vi "CRYConstant Arithmetic Operation.vi"(4 "Constant":dbl, 6 "B data for units":T1={"Name"="", "Curve"=[], "X data"=1, "Y data"=1, "Z data"=1, "X axis"=0, "Y axis"=1, "Z axis"=1, "X unit"="Hz", "Y unit"="", "Z unit"="deg.", "X dB ref"=1.0, "Y dB ref"=1.0, "Z dB ref"=1.0, "single val"=FALSE, "protected"=FALSE, "display X"=TRUE, "display Y"=TRUE, "display Z"=TRUE, "Test Info"="", "Step No."=0, "Plot Settings"={"Color"=0, "Interpolation"=0, "Point Style"=0, "Line Style"=0, "Point Color"=0, "Line Width"=0, "Bar Plot Style"=0, "Fill To"=0}, "AutoProtect"=FALSE} {"Z data" items=["dB", "Lin"]; "X data" items=["dB", "Lin"]; "Y data" items=["dB", "Lin"]; "Z dB ref" format="%.1f"; "Z axis" items=["Log", "Lin"]; "X dB ref" format="%.1f"; "X axis" items=["Log", "Lin"]; "Y axis" items=["Log", "Lin"]; "Y dB ref" format="%.1f"; "Curve"."z" format="%.2f"; "Curve"."y" format="%.2f"; "Curve"."x" format="%.2f"}, 7 "A data for units":T1={"Name"="", "Curve"=[], "X data"=1, "Y data"=1, "Z data"=1, "X axis"=0, "Y axis"=1, "Z axis"=1, "X unit"="Hz", "Y unit"="", "Z unit"="deg.", "X dB ref"=1.0, "Y dB ref"=1.0, "Z dB ref"=1.0, "single val"=FALSE, "protected"=FALSE, "display X"=TRUE, "display Y"=TRUE, "display Z"=TRUE, "Test Info"="", "Step No."=0, "Plot Settings"={"Color"=0, "Interpolation"=0, "Point Style"=0, "Line Style"=0, "Point Color"=0, "Line Width"=0, "Bar Plot Style"=0, "Fill To"=0}, "AutoProtect"=FALSE} {"Z data" items=["dB", "Lin"]; "X data" items=["dB", "Lin"]; "Y data" items=["dB", "Lin"]; "Z dB ref" format="%.1f"; "Z axis" items=["Log", "Lin"]; "X dB ref" format="%.1f"; "X axis" items=["Log", "Lin"]; "Y axis" items=["Log", "Lin"]; "Y dB ref" format="%.1f"; "Curve"."z" format="%.2f"; "Curve"."y" format="%.2f"; "Curve"."x" format="%.2f"}, 8 "B_axis mode":u16(slide) scale=0.0..2.0, 9 "A_axis mode":u16(slide) scale=0.0..2.0, 10 "Work in":u16(slide), 11 "Operator":u16(ring) items=["+", "--", "x", "/"]) -> (3 "Result out":T1={"Name"="", "Curve"=[], "X data"=1, "Y data"=1, "Z data"=1, "X axis"=0, "Y axis"=1, "Z axis"=1, "X unit"="Hz", "Y unit"="", "Z unit"="deg.", "X dB ref"=1.0, "Y dB ref"=1.0, "Z dB ref"=1.0, "single val"=FALSE, "protected"=FALSE, "display X"=TRUE, "display Y"=TRUE, "display Z"=TRUE, "Test Info"="", "Step No."=0, "Plot Settings"={"Color"=0, "Interpolation"=0, "Point Style"=0, "Line Style"=0, "Point Color"=0, "Line Width"=0, "Bar Plot Style"=0, "Fill To"=0}, "AutoProtect"=FALSE} {"Z data" items=["dB", "Lin"]; "X data" items=["dB", "Lin"]; "Y data" items=["dB", "Lin"]; "Z dB ref" format="%.1f"; "Z axis" items=["Log", "Lin"]; "X dB ref" format="%.1f"; "X axis" items=["Log", "Lin"]; "Y axis" items=["Log", "Lin"]; "Y dB ref" format="%.1f"; "Curve"."z" format="%.2f"; "Curve"."y" format="%.2f"; "Curve"."x" format="%.2f"})   [LabVIEW 2013]
uses:
  Typedef Control/CRYData Cluster.ctl
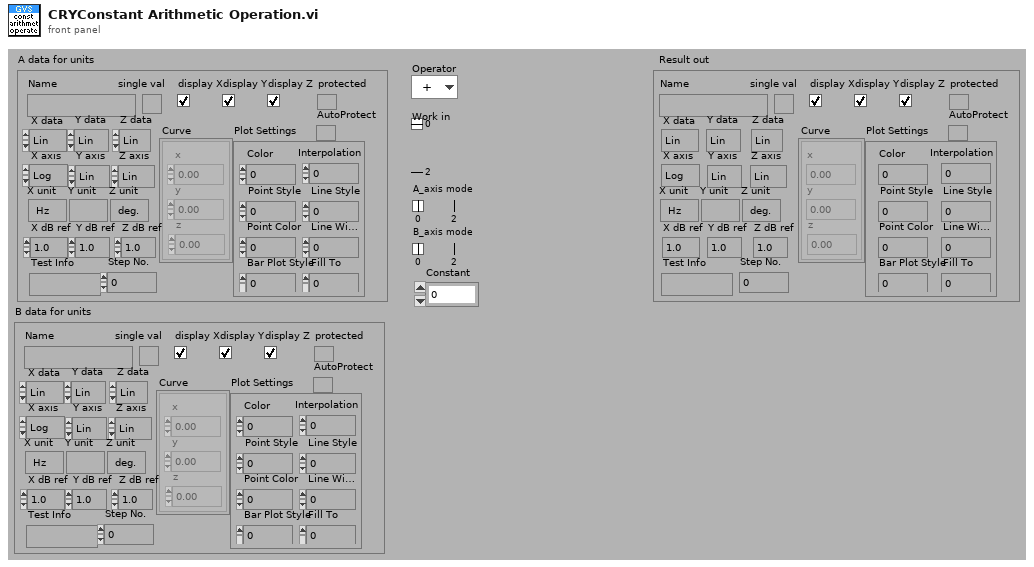
[diagram p1: front panel]
types:
  T1 = typedef "CRYData Cluster.ctl" = cluster{"Name":string, "Curve":cluster{"x":dbl, "y":dbl, "z":dbl}[], "X data":u16, "Y data":u16, "Z data":u16, "X axis":u16, "Y axis":u16, "Z axis":u16, "X unit":string, "Y unit":string, "Z unit":string, "X dB ref":dbl, "Y dB ref":dbl, "Z dB ref":dbl, "single val":bool, "protected":bool, "display X":bool, "display Y":bool, "display Z":bool, "Test Info":string, "Step No.":i32, "Plot Settings":cluster{"Color":u32, "Interpolation":u8, "Point Style":u8, "Line Style":u8, "Point Color":u32, "Line Width":u8, "Bar Plot Style":u8, "Fill To":i16}, "AutoProtect":bool}
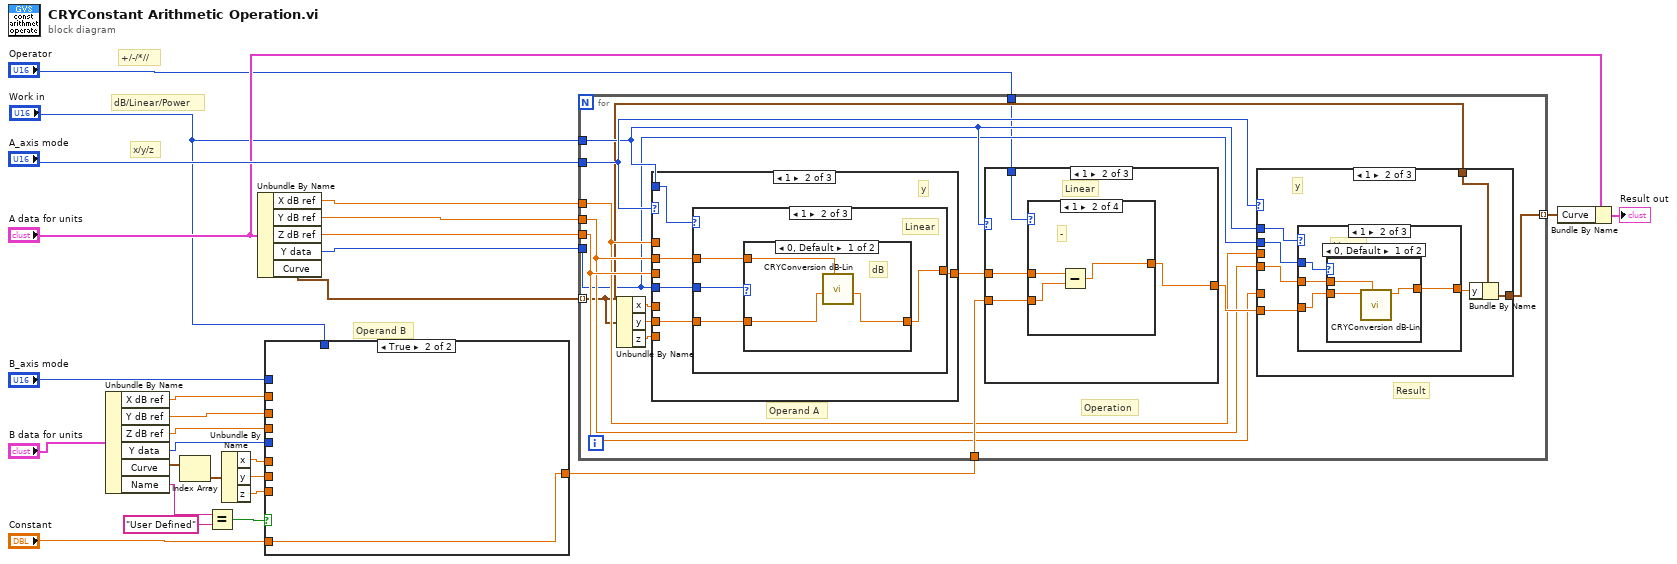
[diagram p0: block diagram]
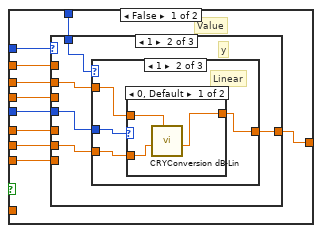
[diagram p2: hidden frame]
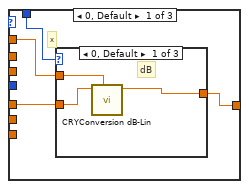
[diagram p3: hidden frame]
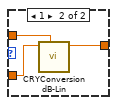
[diagram p7: hidden frame]
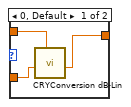
[diagram p10: hidden frame]
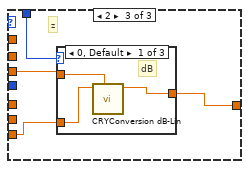
[diagram p11: hidden frame]
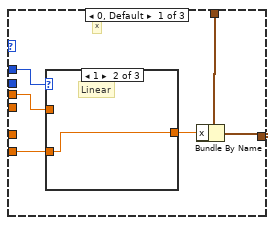
[diagram p14: hidden frame]
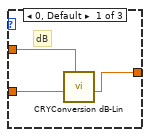
[diagram p15: hidden frame]
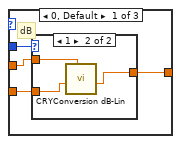
[diagram p17: hidden frame]
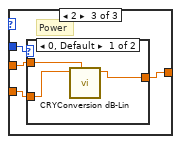
[diagram p20: hidden frame]
diagram:
  # "Operand B"
  # "+/-/*//"
  # "dB/Linear/Power"
  # "x/y/z"
  n1 = Unbundle By Name("B data for units") -> ("X dB ref"=w19:dbl, "Y dB ref"=w18:dbl, "Z dB ref"=w17:dbl, "Y data"=w16:u16, "Curve"=w14:cluster{"x":dbl, "y":dbl, "z":dbl}[], "Name"=w21:string)
  n2 = Index Array(array=w14) -> (element=w15:cluster{"x":dbl, "y":dbl, "z":dbl})  [unwired: 1 in]
  n3 = Equal?(x=w21, y="User Defined") -> (x = y?=w20:bool)
  n4 = Unbundle By Name(w15) -> ("x"=w13:dbl, "y"=w12:dbl, "z"=w11:dbl)
  n5 = Unbundle By Name("A data for units") -> ("X dB ref"=w27:dbl, "Y dB ref"=w26:dbl, "Z dB ref"=w25:dbl, "Y data"=w24:u16, "Curve"=w23:cluster{"x":dbl, "y":dbl, "z":dbl}[])
  n6 = case shown="True" w20 {
    tunnel: "Constant" -> [_ w85]
    tunnel: "B_axis mode" -> [w37 _]
    tunnel: w19 -> [w31 _]
    tunnel: w18 -> [w30 _]
    tunnel: w17 -> [w29 _]
    tunnel: w16 -> [w28 _]
    tunnel: w13 -> [w36 _]
    tunnel: w12 -> [w34 _]
    tunnel: w11 -> [w33 _]
    tunnel: [w35 w85] -> w10
    tunnel: "Work in" -> [w32 _]
    frame False {
      # "Value"
      n7 = case shown="1" w37 {
        tunnel: [w38 w48 w76] -> w35
        tunnel: w36 -> [w39 _ _]
        tunnel: w34 -> [_ w50 _]
        tunnel: w33 -> [_ _ w77]
        tunnel: w32 -> [w40 w49 w79]
        tunnel: w31 -> [w41 _ _]
        tunnel: w30 -> [_ w51 _]
        tunnel: w29 -> [_ _ w78]
        tunnel: w28 -> [_ w47 _]
        frame 0, Default {
          # "x"
          n8 = case shown="0, Default" w40 {
            tunnel: w41 -> [w44 _ _]
            tunnel: w39 -> [w43 w45 w46]
            tunnel: [w42 w45 w46] -> w38
            frame 0, Default {
              # "dB"
              n9 = call "CRYConversion dB-Lin.vi"("dB ref."=w44, "Lin In"=w43) -> ("Log Out"=w42:dbl)  [unwired: 4 in, 3 out]
            }
            frame 1 {
              # "Linear"
            }
            frame 2 {
              # "Power"
            }
          }
        }
        frame 1 {
          # "y"
          n10 = case shown="1" w49 {
            tunnel: w51 -> [w52 w61 w71]
            tunnel: w50 -> [w54 w62 w69]
            tunnel: [w53 w60 w68] -> w48
            tunnel: w47 -> [w55 w63 w70]
            frame 0, Default {
              # "dB"
              n11 = case shown="0, Default" w55 {
                tunnel: [w56 w57] -> w53
                tunnel: w54 -> [w56 w58]
                tunnel: w52 -> [_ w59]
                frame 0, Default {
                }
                frame 1 {
                  n12 = call "CRYConversion dB-Lin.vi"("dB ref."=w59, "Lin In"=w58) -> ("Log Out"=w57:dbl)  [unwired: 4 in, 3 out]
                }
              }
            }
            frame 1 {
              # "Linear"
              n13 = case shown="0, Default" w63 {
                tunnel: [w64 w67] -> w60
                tunnel: w62 -> [w65 w67]
                tunnel: w61 -> [w66 _]
                frame 0, Default {
                  n14 = call "CRYConversion dB-Lin.vi"("dB ref."=w66, "Log In"=w65) -> ("Lin Out"=w64:dbl)  [unwired: 4 in, 3 out]
                }
                frame 1 {
                }
              }
            }
            frame 2 {
              # "Power"
              n15 = case shown="1" w70 {
                tunnel: [w73 w75] -> w68
                tunnel: w69 -> [w72 w75]
                tunnel: w71 -> [w74 _]
                frame 0, Default {
                  n16 = call "CRYConversion dB-Lin.vi"("dB ref."=w74, "Log In"=w72) -> ("Lin Out"=w73:dbl)  [unwired: 4 in, 3 out]
                }
                frame 1 {
                }
              }
            }
          }
        }
        frame 2 {
          # "z"
          n17 = case shown="0, Default" w79 {
            tunnel: w78 -> [w82 _ _]
            tunnel: w77 -> [w81 w83 w84]
            tunnel: [w80 w83 w84] -> w76
            frame 0, Default {
              # "dB"
              n18 = call "CRYConversion dB-Lin.vi"("dB ref."=w82, "Lin In"=w81) -> ("Log Out"=w80:dbl)  [unwired: 4 in, 3 out]
            }
            frame 1 {
              # "Linear"
            }
            frame 2 {
              # "Power"
            }
          }
        }
      }
    }
    frame True {
    }
  }
  n19 = for {
    tunnel: "A_axis mode" -> [w95]
    tunnel: "Work in" -> [w94]
    tunnel: w27 -> [w90]
    tunnel: w26 -> [w91]
    tunnel: w25 -> [w92]
    tunnel: w24 -> [w87]
    tunnel: w23 -> [w88] mode=indexing
    tunnel: "Operator" -> [w86]
    tunnel: w10 -> [w96]
    tunnel: [w89] -> w5 mode=indexing
    # "Result"
    # "Operation"
    # "Operand A"
    n20 = Unbundle By Name(w88) -> ("x"=w100:dbl, "y"=w99:dbl, "z"=w98:dbl)
    n21 = case shown="1" w95 {
      tunnel: w94 -> [w211 w221 w246]
      tunnel: w90 -> [w210 _ _]
      tunnel: w91 -> [_ w217 _]
      tunnel: w92 -> [_ _ w248]
      tunnel: w87 -> [_ w220 _]
      tunnel: w100 -> [w209 _ _]
      tunnel: w99 -> [_ w219 _]
      tunnel: w98 -> [_ _ w249]
      tunnel: [w208 w218 w247] -> w97
      frame 0, Default {
        # "x"
        n22 = case shown="0, Default" w211 {
          tunnel: w210 -> [w214 _ _]
          tunnel: w209 -> [w213 w215 w216]
          tunnel: [w212 w215 w216] -> w208
          frame 0, Default {
            # "dB"
            n23 = call "CRYConversion dB-Lin.vi"("dB ref."=w214, "Lin In"=w213) -> ("Log Out"=w212:dbl)  [unwired: 4 in, 3 out]
          }
          frame 1 {
            # "Linear"
          }
          frame 2 {
            # "Power"
          }
        }
      }
      frame 1 {
        # "y"
        n24 = case shown="1" w221 {
          tunnel: [w223 w231 w238] -> w218
          tunnel: w220 -> [w225 w230 w240]
          tunnel: w219 -> [w224 w232 w239]
          tunnel: w217 -> [w222 w233 w241]
          frame 0, Default {
            # "dB"
            n25 = case shown="1" w225 {
              tunnel: w224 -> [w226 w228]
              tunnel: [w226 w227] -> w223
              tunnel: w222 -> [_ w229]
              frame 0, Default {
                # "dB"
              }
              frame 1 {
                # "Linear"
                n26 = call "CRYConversion dB-Lin.vi"("dB ref."=w229, "Lin In"=w228) -> ("Log Out"=w227:dbl)  [unwired: 4 in, 3 out]
              }
            }
          }
          frame 1 {
            # "Linear"
            n27 = case shown="0, Default" w230 {
              tunnel: w232 -> [w235 w237]
              tunnel: [w234 w237] -> w231
              tunnel: w233 -> [w236 _]
              frame 0, Default {
                # "dB"
                n28 = call "CRYConversion dB-Lin.vi"("dB ref."=w236, "Log In"=w235) -> ("Lin Out"=w234:dbl)  [unwired: 4 in, 3 out]
              }
              frame 1 {
                # "Linear"
              }
            }
          }
          frame 2 {
            # "Power"
            n29 = case shown="0, Default" w240 {
              tunnel: w239 -> [w243 w245]
              tunnel: [w242 w245] -> w238
              tunnel: w241 -> [w244 _]
              frame 0, Default {
                # "dB"
                n30 = call "CRYConversion dB-Lin.vi"("dB ref."=w244, "Log In"=w243) -> ("Lin Out"=w242:dbl)  [unwired: 4 in, 3 out]
              }
              frame 1 {
                # "Linear"
              }
            }
          }
        }
      }
      frame 2 {
        # "z"
        n31 = case shown="2" w246 {
          tunnel: w248 -> [w252 _ _]
          tunnel: w249 -> [w251 w253 w254]
          tunnel: [w250 w253 w254] -> w247
          frame 0, Default {
            # "dB"
            n32 = call "CRYConversion dB-Lin.vi"("dB ref."=w252, "Lin In"=w251) -> ("Log Out"=w250:dbl)  [unwired: 4 in, 3 out]
          }
          frame 1 {
            # "Linear"
          }
          frame 2 {
            # "Power"
          }
        }
      }
    }
    n33 = case shown="1" w94 {
      tunnel: w86 -> [w158 w168 w184]
      tunnel: w97 -> [w157 w167 w183]
      tunnel: w96 -> [w156 w166 w182]
      tunnel: [w155 w165 w181] -> w93
      frame 0, Default {
        # "dB"
        n34 = case shown="0, Default" w158 {
          tunnel: w157 -> [w161 w164]
          tunnel: w156 -> [w160 w163]
          tunnel: [w159 w162] -> w155
          frame 0, Default {
            # "+"
            n35 = Add(x=w161, y=w160) -> (x+y=w159:dbl)
          }
          frame 1 {
            # "-"
            n36 = Subtract(x=w164, y=w163) -> (x-y=w162:dbl)
          }
        }
      }
      frame 1 {
        # "Linear"
        n37 = case shown="1" w168 {
          tunnel: w167 -> [w171 w174 w175 w180]
          tunnel: w166 -> [w170 w173 w177 w179]
          tunnel: [w169 w172 w176 w178] -> w165
          frame 0, Default {
            # "+"
            n38 = Add(x=w171, y=w170) -> (x+y=w169:dbl)
          }
          frame 1 {
            # "-"
            n39 = Subtract(x=w174, y=w173) -> (x-y=w172:dbl)
          }
          frame 2 {
            # "*"
            n40 = Multiply(x=w175, y=w177) -> (x*y=w176:dbl)
          }
          frame 3 {
            # "/"
            n41 = Divide(x=w180, y=w179) -> (x/y=w178:dbl)
          }
        }
      }
      frame 2 {
        # "Power"
        n42 = case shown="3" w184 {
          tunnel: w183 -> [w190 w197 w200 w205]
          tunnel: w182 -> [w189 w196 w202 w207]
          tunnel: [w185 w191 w201 w206] -> w181
          frame 0, Default {
            # "+"
            n43 = Square(x=w190) -> (x^2=w188:dbl)
            n44 = Square(x=w189) -> (x^2=w187:dbl)
            n45 = Add(x=w188, y=w187) -> (x+y=w186:dbl)
            n46 = Square Root(x=w186) -> (sqrt(x)=w185:dbl)
          }
          frame 1 {
            # "-"
            n47 = Square(x=w197) -> (x^2=w195:dbl)
            n48 = Square(x=w196) -> (x^2=w194:dbl)
            n49 = Subtract(x=w195, y=w194) -> (x-y=w193:dbl)
            n50 = Absolute Value(x=w193) -> (abs(x)=w192:dbl)
            n51 = Square Root(x=w192) -> (sqrt(x)=w191:dbl)
          }
          frame 2 {
            # "*"
            n52 = Absolute Value(x=w202) -> (abs(x)=w198:dbl)
            n53 = Square Root(x=w198) -> (sqrt(x)=w199:dbl)
            n54 = Multiply(x=w200, y=w199) -> (x*y=w201:dbl)
          }
          frame 3 {
            # "/"
            n55 = Absolute Value(x=w207) -> (abs(x)=w203:dbl)
            n56 = Square Root(x=w203) -> (sqrt(x)=w204:dbl)
            n57 = Divide(x=w205, y=w204) -> (x/y=w206:dbl)
          }
        }
      }
    }
    n58 = case shown="1" w95 {
      tunnel: [w101 w112 w146] -> w89
      tunnel: w94 -> [w106 w118 w145]
      tunnel: w93 -> [w105 w117 w149]
      tunnel: w92 -> [_ _ w148]
      tunnel: w91 -> [_ w116 _]
      tunnel: w90 -> [w104 _ _]
      tunnel: w88 -> [w102 w115 w147]
      tunnel: w87 -> [_ w114 _]
      frame 0, Default {
        # "x"
        n59 = case shown="1" w106 {
          tunnel: [w108 w110 w111] -> w103
          tunnel: w105 -> [w109 w110 w111]
          tunnel: w104 -> [w107 _ _]
          frame 0, Default {
            # "dB"
            n60 = call "CRYConversion dB-Lin.vi"("dB ref."=w107, "Log In"=w109) -> ("Lin Out"=w108:dbl)  [unwired: 4 in, 3 out]
          }
          frame 1 {
            # "Linear"
          }
          frame 2 {
            # "Power"
          }
        }
        n61 = Bundle By Name(cluster=w102, "x"=w103) -> (w101:cluster{"x":dbl, "y":dbl, "z":dbl})
      }
      frame 1 {
        # "y"
        n62 = case shown="1" w118 {
          tunnel: [w120 w127 w137] -> w113
          tunnel: w117 -> [w121 w128 w138]
          tunnel: w116 -> [w119 w129 w136]
          tunnel: w114 -> [w122 w130 w135]
          frame 0, Default {
            # "dB"
            n63 = case shown="1" w122 {
              tunnel: [w123 w124] -> w120
              tunnel: w121 -> [w123 w125]
              tunnel: w119 -> [_ w126]
              frame 0, Default {
              }
              frame 1 {
                n64 = call "CRYConversion dB-Lin.vi"("dB ref."=w126, "Log In"=w125) -> ("Lin Out"=w124:dbl)  [unwired: 4 in, 3 out]
              }
            }
          }
          frame 1 {
            # "Linear"
            n65 = case shown="0, Default" w130 {
              tunnel: w129 -> [w133 _]
              tunnel: w128 -> [w132 w134]
              tunnel: [w131 w134] -> w127
              frame 0, Default {
                n66 = call "CRYConversion dB-Lin.vi"("dB ref."=w133, "Lin In"=w132) -> ("Log Out"=w131:dbl)  [unwired: 4 in, 3 out]
              }
              frame 1 {
              }
            }
          }
          frame 2 {
            # "Power"
            n67 = case shown="0, Default" w135 {
              tunnel: [w139 w142] -> w137
              tunnel: w138 -> [w140 w142]
              tunnel: w136 -> [w141 _]
              frame 0, Default {
                n68 = call "CRYConversion dB-Lin.vi"("dB ref."=w141, "Lin In"=w140) -> ("Log Out"=w139:dbl)  [unwired: 4 in, 3 out]
              }
              frame 1 {
              }
            }
          }
        }
        n69 = Bundle By Name(cluster=w115, "y"=w113) -> (w112:cluster{"x":dbl, "y":dbl, "z":dbl})
      }
      frame 2 {
        # "z"
        n70 = case shown="0, Default" w145 {
          tunnel: [w152 w153 w154] -> w144
          tunnel: w149 -> [w151 w153 w154]
          tunnel: w148 -> [w150 _ _]
          frame 0, Default {
            # "dB"
            n71 = call "CRYConversion dB-Lin.vi"("dB ref."=w150, "Log In"=w151) -> ("Lin Out"=w152:dbl)  [unwired: 4 in, 3 out]
          }
          frame 1 {
            # "Linear"
          }
          frame 2 {
            # "Power"
          }
        }
        n72 = call "CRYLowUp360to180.vi"("Value In"=w144) -> ("Value Out"=w143:dbl)  [unwired: 10 in]
        n73 = Bundle By Name(cluster=w147, "z"=w143) -> (w146:cluster{"x":dbl, "y":dbl, "z":dbl})
      }
    }
  }
  n74 = Bundle By Name(cluster="A data for units", "Curve"=w5) -> (→"Result out":T1)
